vi "Calculator.vi"() -> ()   [LabVIEW 2014]
panel:
  in  "stop":bool
  out "Calculator Display":string
  in  "Calculator":T1
  # "Calculator"
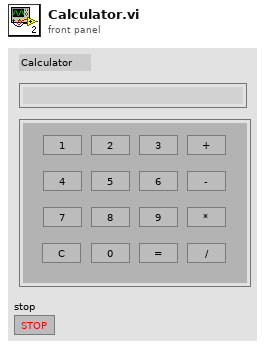
[diagram p1: front panel]
types:
  T1 = cluster{"0":bool, "1":bool, "2":bool, "3":bool, "4":bool, "5":bool, "6":bool, "7":bool, "8":bool, "9":bool, "C":bool, "=":bool, "+":bool, "-":bool, "*":bool, "/":bool}
  T2 = enum16{"no function", "add", "sub", "mul", "divide"}
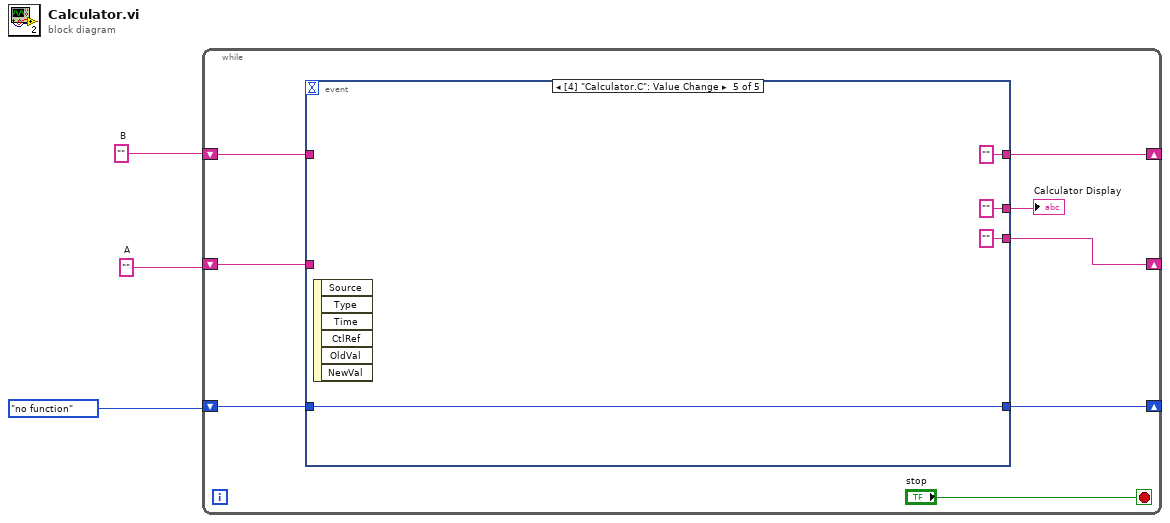
[diagram p0: block diagram]
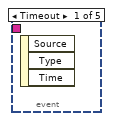
[diagram p2: hidden frame]
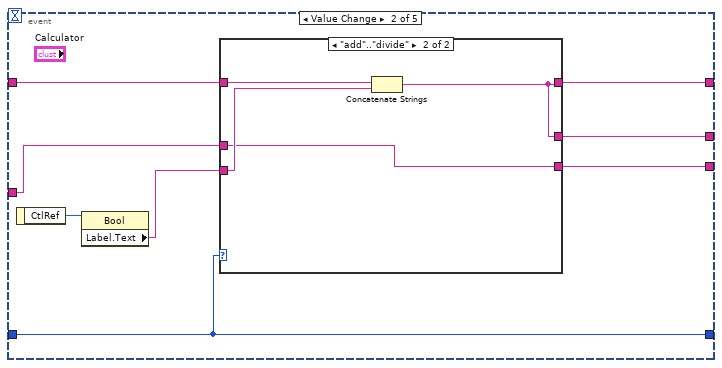
[diagram p3: hidden frame]
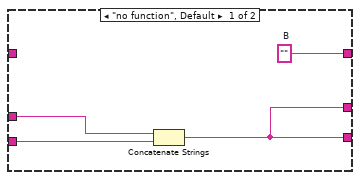
[diagram p4: hidden frame]
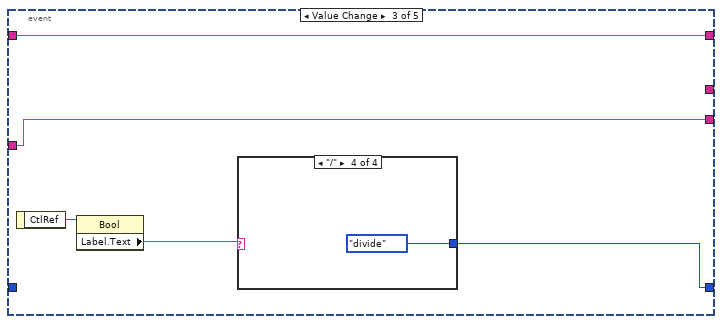
[diagram p5: hidden frame]
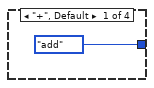
[diagram p6: hidden frame]
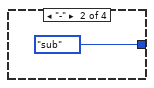
[diagram p7: hidden frame]
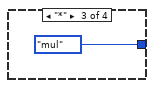
[diagram p8: hidden frame]
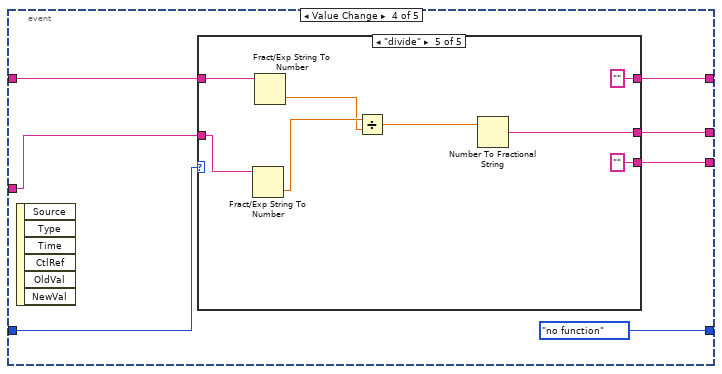
[diagram p9: hidden frame]
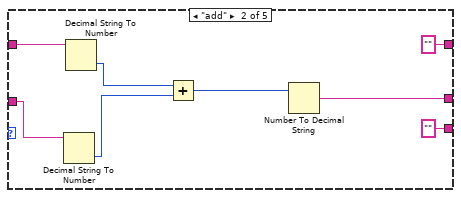
[diagram p11: hidden frame]
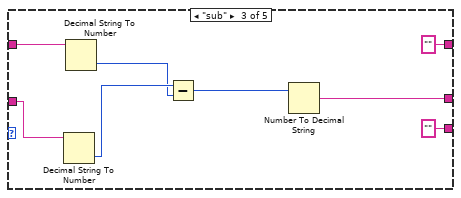
[diagram p12: hidden frame]
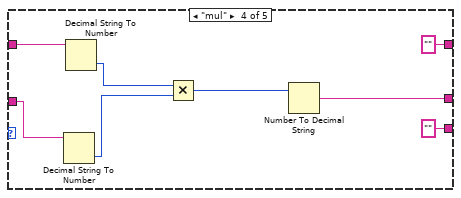
[diagram p13: hidden frame]
diagram:
  w2 = ""  # A
  w3 = ""  # B
  n1 = while {
    shift-right: [w6] -> _
    shift-left: w3 -> [w11]
    shift-right: [w7] -> _
    shift-left: w2 -> [w10]
    shift-right: [w8] -> _
    shift-left: T2."no function" -> [w9]
    stop <- "stop" stop-if-true
    n2 = event shown="[4] \"Calculator.C\": Value Change" {
      selector: _ -> [_ _ _ _ _]
      dyn-events: _ -> [_ _ _ _ _]
      timeout: _ -> [_ _ _ _ _]
      tunnel: w11 -> [_ w13 w32 w43 _]
      tunnel: w10 -> [_ w16 w31 w42 _]
      tunnel: w9 -> [_ w18 _ w38 w81]
      tunnel: [_ w18 w28 T2."no function" w81] -> w8
      tunnel: [_ w15 w31 w40 "" ("A")] -> w7
      tunnel: [_ w14 w32 w41 "" ("B")] -> w6
      tunnel: [_ w12 _ w39 "" ("A")] -> w5
      event Timeout {
        n3 = event-data() -> ()  [unwired: 1 in, 3 out]
      }
      event "Calculator.1", "Calculator.2", "Calculator.3", "Calculator.4", "Calculator.5", "Calculator.6", "Calculator.7", "Calculator.8", "Calculator.9": Value Change {
        n4 = event-data() -> ("CtlRef"=w19:refnum<vi>)  [unwired: 1 in]
        n5 = property class="Bool"(reference=w19) -> ("Label.Text"=w17:string)  [unwired: 1 in, 2 out]
        n6 = case shown="\"add\"..\"divide\"" w18 {
          tunnel: w17 -> [w23 w26]
          tunnel: w16 -> [w22 w24]
          tunnel: [w20 w24] -> w15
          tunnel: [w21 w25] -> w14
          tunnel: w13 -> [_ w27]
          tunnel: [w20 w25] -> w12
          frame "no function", Default {
            w21 = ""  # B
            n7 = Concatenate Strings(w22, w23) -> (w20:string)
          }
          frame "add".."divide" {
            n8 = Concatenate Strings(w27, w26) -> (w25:string)
          }
        }
      }
      event "Calculator.+", "Calculator.-", "Calculator.*", "Calculator./": Value Change {
        n9 = event-data() -> ("CtlRef"=w30:refnum<vi>)  [unwired: 1 in]
        n10 = property class="Bool"(reference=w30) -> ("Label.Text"=w29:string)  [unwired: 1 in, 2 out]
        n11 = case shown="\"/\"" w29 {
          tunnel: [T2."add" T2."sub" T2."mul" T2."divide"] -> w28
          frame "+", Default {
          }
          frame "-" {
          }
          frame "*" {
          }
          frame "/" {
          }
        }
      }
      event "Calculator.=": Value Change {
        n12 = event-data() -> ()  [unwired: 1 in, 6 out]
        n13 = case shown="\"divide\"" w38 {
          tunnel: w43 -> [w45 w53 w61 w69 w77]
          tunnel: w42 -> [w44 w51 w60 w67 w76]
          tunnel: [w45 "" ("B") "" ("B") "" ("B") "" ("B")] -> w41
          tunnel: [w44 "" ("A") "" ("A") "" ("A") "" ("A")] -> w40
          tunnel: [w44 w48 w58 w64 w74] -> w39
          frame "no function", Default {
          }
          frame "add" {
            n14 = Decimal String To Number(string=w51) -> (number=w50:i32)  [unwired: 2 in, 1 out]
            n15 = Decimal String To Number(string=w53) -> (number=w52:i32)  [unwired: 2 in, 1 out]
            n16 = Add(x=w52, y=w50) -> (x+y=w49:i32)
            n17 = Number To Decimal String(number=w49) -> (decimal integer string=w48:string)  [unwired: 1 in]
          }
          frame "sub" {
            n18 = Decimal String To Number(string=w60) -> (number=w55:i32)  [unwired: 2 in, 1 out]
            n19 = Decimal String To Number(string=w61) -> (number=w54:i32)  [unwired: 2 in, 1 out]
            n20 = Subtract(x=w55, y=w54) -> (x-y=w59:i32)
            n21 = Number To Decimal String(number=w59) -> (decimal integer string=w58:string)  [unwired: 1 in]
          }
          frame "mul" {
            n22 = Decimal String To Number(string=w67) -> (number=w66:i32)  [unwired: 2 in, 1 out]
            n23 = Decimal String To Number(string=w69) -> (number=w68:i32)  [unwired: 2 in, 1 out]
            n24 = Multiply(x=w68, y=w66) -> (x*y=w65:i32)
            n25 = Number To Decimal String(number=w65) -> (decimal integer string=w64:string)  [unwired: 1 in]
          }
          frame "divide" {
            n26 = Fract/Exp String To Number(string=w76) -> (number=w71:dbl)  [unwired: 3 in, 1 out]
            n27 = Fract/Exp String To Number(string=w77) -> (number=w70:dbl)  [unwired: 3 in, 1 out]
            n28 = Divide(x=w71, y=w70) -> (x/y=w75:dbl)
            n29 = Number To Fractional String(number=w75) -> (F-format string=w74:string)  [unwired: 3 in]
          }
        }
      }
      event "Calculator.C": Value Change {
        n30 = event-data() -> ()  [unwired: 1 in, 6 out]
      }
    }
    "Calculator Display" <- w5
  }
